vi "Command.vi"(8 "error in":errorcluster, 10 "connection ID":refnum<k5>, 11 "Command":string) -> (0 "Dbl_out":dbl, 1 "Error":bool, 2 "connection ID 2":refnum<k5>, 3 "data out":string, 4 "error out":errorcluster, 5 "Hardware Error":bool)   [LabVIEW 2018]
panel:
  out "bytes written":i32
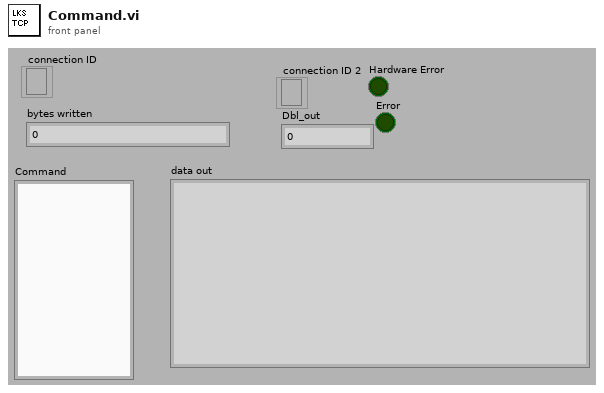
[diagram p1: front panel]
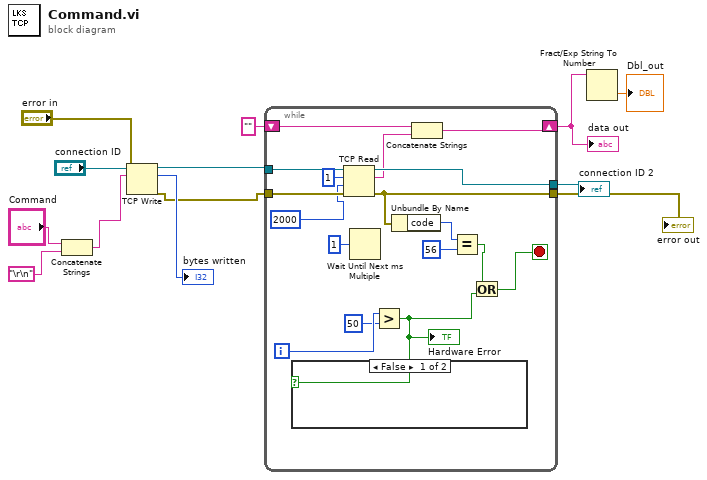
[diagram p0: block diagram]
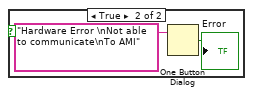
[diagram p2: hidden frame]
diagram:
  n1 = Concatenate Strings("Command", "\r\n") -> (w9:string)
  n2 = TCP Write(connection ID="connection ID", data in=w9, error in (no error)="error in") -> (connection ID out=w12:refnum<k5>, bytes written=→"bytes written":i32, error out=w11:errorcluster)  [unwired: 1 out]
  n3 = while {
    tunnel: w12 -> [w30]
    tunnel: w11 -> [w29]
    tunnel: [w27] -> w5
    tunnel: [w25] -> w1
    shift-right: [w22] -> w4
    shift-left: "" -> [w20]
    i -> [w18]
    stop <- w15 stop-if-true
    n4 = TCP Read(connection ID=w30, bytes to read=1, error in (no error)=w29, 9:2000 ("timeout ms (25000)")) -> (connection ID out=w27:refnum<k5>, data out=w21:string, error out=w25:errorcluster)  [unwired: 1 out]
    n5 = Wait Until Next ms Multiple(millisecond multiple=u32 1) -> ()  [unwired: 1 out]
    n6 = Greater?(x=w18, y=50) -> (0:w14:bool)
    "Hardware Error" <- w14
    n7 = case shown="False" w14 {
      frame False {
      }
      frame True {
        n8 = One Button Dialog(message="Hardware Error \nNot able to communicate\nTo AMI") -> (true=→"Error":bool)  [unwired: 1 in]
      }
    }
    n9 = Unbundle By Name(w25) -> ("code"=w24:i32)
    n10 = Concatenate Strings(w20, w21) -> (w22:string)
    n11 = Equal?(x=w24, y=56) -> (x = y?=w16:bool)
    n12 = Or(x=w16, y=w14) -> (x .or. y?=w15:bool)
  }
  "data out" <- w4
  "connection ID 2" <- w5
  "error out" <- w1
  n13 = Fract/Exp String To Number(string=w4) -> (number=→"Dbl_out":dbl)  [unwired: 4 out]
